vi "Vision Update Time.vi"() -> ()   [LabVIEW 2025]
uses:
  <vilib>/Rock Robotics/Network Tables/NT Write Number.vi
panel:
  out "Vision Time":dbl
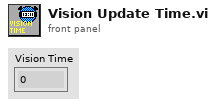
[diagram p1: front panel]
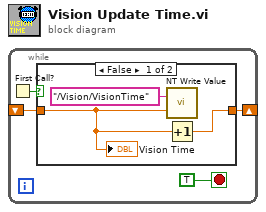
[diagram p0: block diagram]
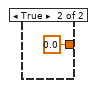
[diagram p2: hidden frame]
diagram:
  n1 = while {
    shift-right: [w1] -> _
    shift-left: _ -> [w2]
    stop <- TRUE stop-if-true
    n2 = First Call?() -> (First Call?: T/F=w3:bool)
    n3 = case shown="False" w3 {
      tunnel: w2 -> [w6 _]
      tunnel: [w5 0.0] -> w1
      frame False {
        n4 = call-poly <vilib>:"NT Write Value.vi"("value"=w6, "name"="/Vision/VisionTime" ("Name")) -> ()  [unwired: 9 in, 1 out]
        n5 = Increment(x=w6) -> (x+1=w5:dbl)
        "Vision Time" <- w6
      }
      frame True {
      }
    }
  }
